vi "Plugin Post-Build Action.vi"(5 "Files Generated by Build":path[](array[path]), 6 "Top Level/Always Included VIs":path[](array[path]), 7 "Destination Path":path, 8 "error in (no error)":errorcluster, 9 "Target Name":string, 10 "Build Specification Name":string, 11 "Project Path":path) -> (0 "error out":errorcluster)   [LabVIEW 2019]
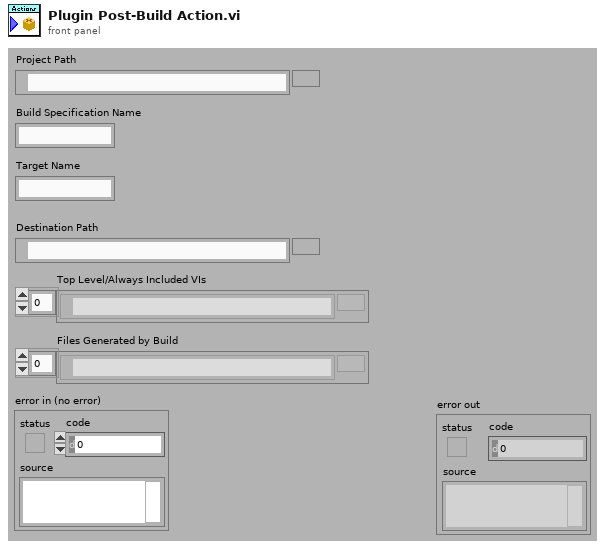
[diagram p1: front panel]
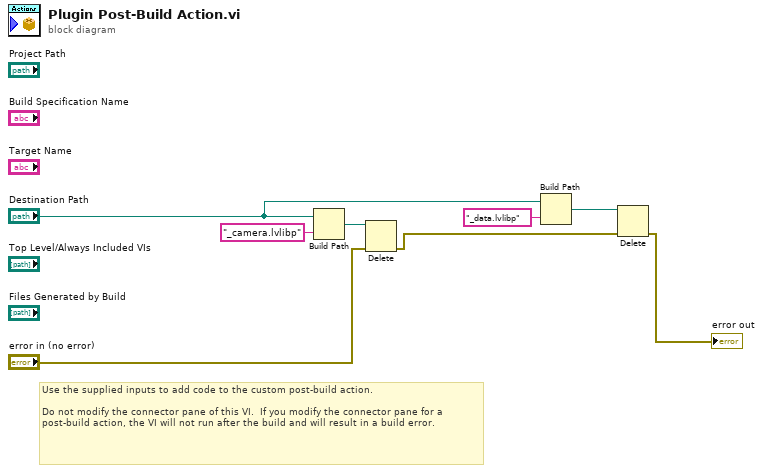
[diagram p0: block diagram]
diagram:
  # "Use the supplied inputs to add code to the custom post-build action.\n\nDo not modify the connector pane of this VI.  If you modify the connector pane for a post-build action, the VI will not run after the build and will result in a build error."
  n1 = Build Path(base path="Destination Path", name or relative path="_camera.lvlibp") -> (appended path=w7:path)
  n2 = Delete(path (use dialog)=w7, error in="error in (no error)") -> (error out=w2:errorcluster)  [unwired: 3 in, 2 out]
  n3 = Build Path(base path="Destination Path", name or relative path="_data.lvlibp") -> (appended path=w3:path)
  n4 = Delete(path (use dialog)=w3, error in=w2) -> (error out=→"error out":errorcluster)  [unwired: 3 in, 2 out]
